vi "Dig Target.vi"() -> ()   [LabVIEW 2018, in "Tests.lvlib" / "Toolkit.lvlib"]
uses:
  Toolkit.lvlib
panel:
  in  "Input":bool[](array[boolean])=[FALSE, FALSE, FALSE, TRUE, FALSE, FALSE]
  out "Any?":bool
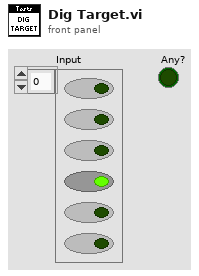
[diagram p1: front panel]
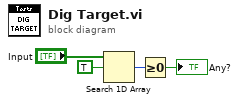
[diagram p0: block diagram]
diagram:
  n1 = Search 1D Array(1D array="Input", element=TRUE) -> (index of element=w1:i32)  [unwired: 1 in]
  n2 = Greater Or Equal To 0?(x=w1) -> (x >= 0?=→"Any?":bool)
